vi "Practica02.vi"() -> ()   [LabVIEW 2021]
uses:
  <vilib>/DAQmx/configure/timing.llb/DAQmx Timing (Sample Clock).vi
  <vilib>/DAQmx/create/channels.llb/DAQmx Create Channel (DI-Digital Input).vi
  <vilib>/DAQmx/read.llb/DAQmx Read (Digital 1D Bool 1Chan 1Samp).vi
  <vilib>/Utility/file.llb/Write Delimited Spreadsheet (DBL).vi
panel:
  out "Numero":u32
  out "appended array":bool[](array[boolean])
  in  "stop":bool
  out "Slide":dbl(slide) scale=0.0..1.0
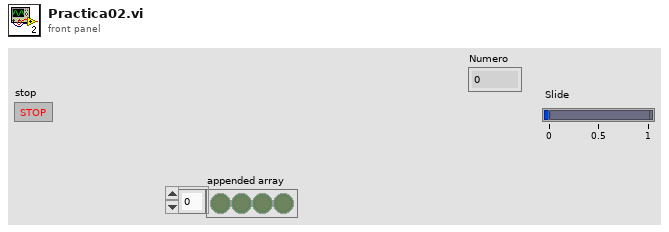
[diagram p1: front panel]
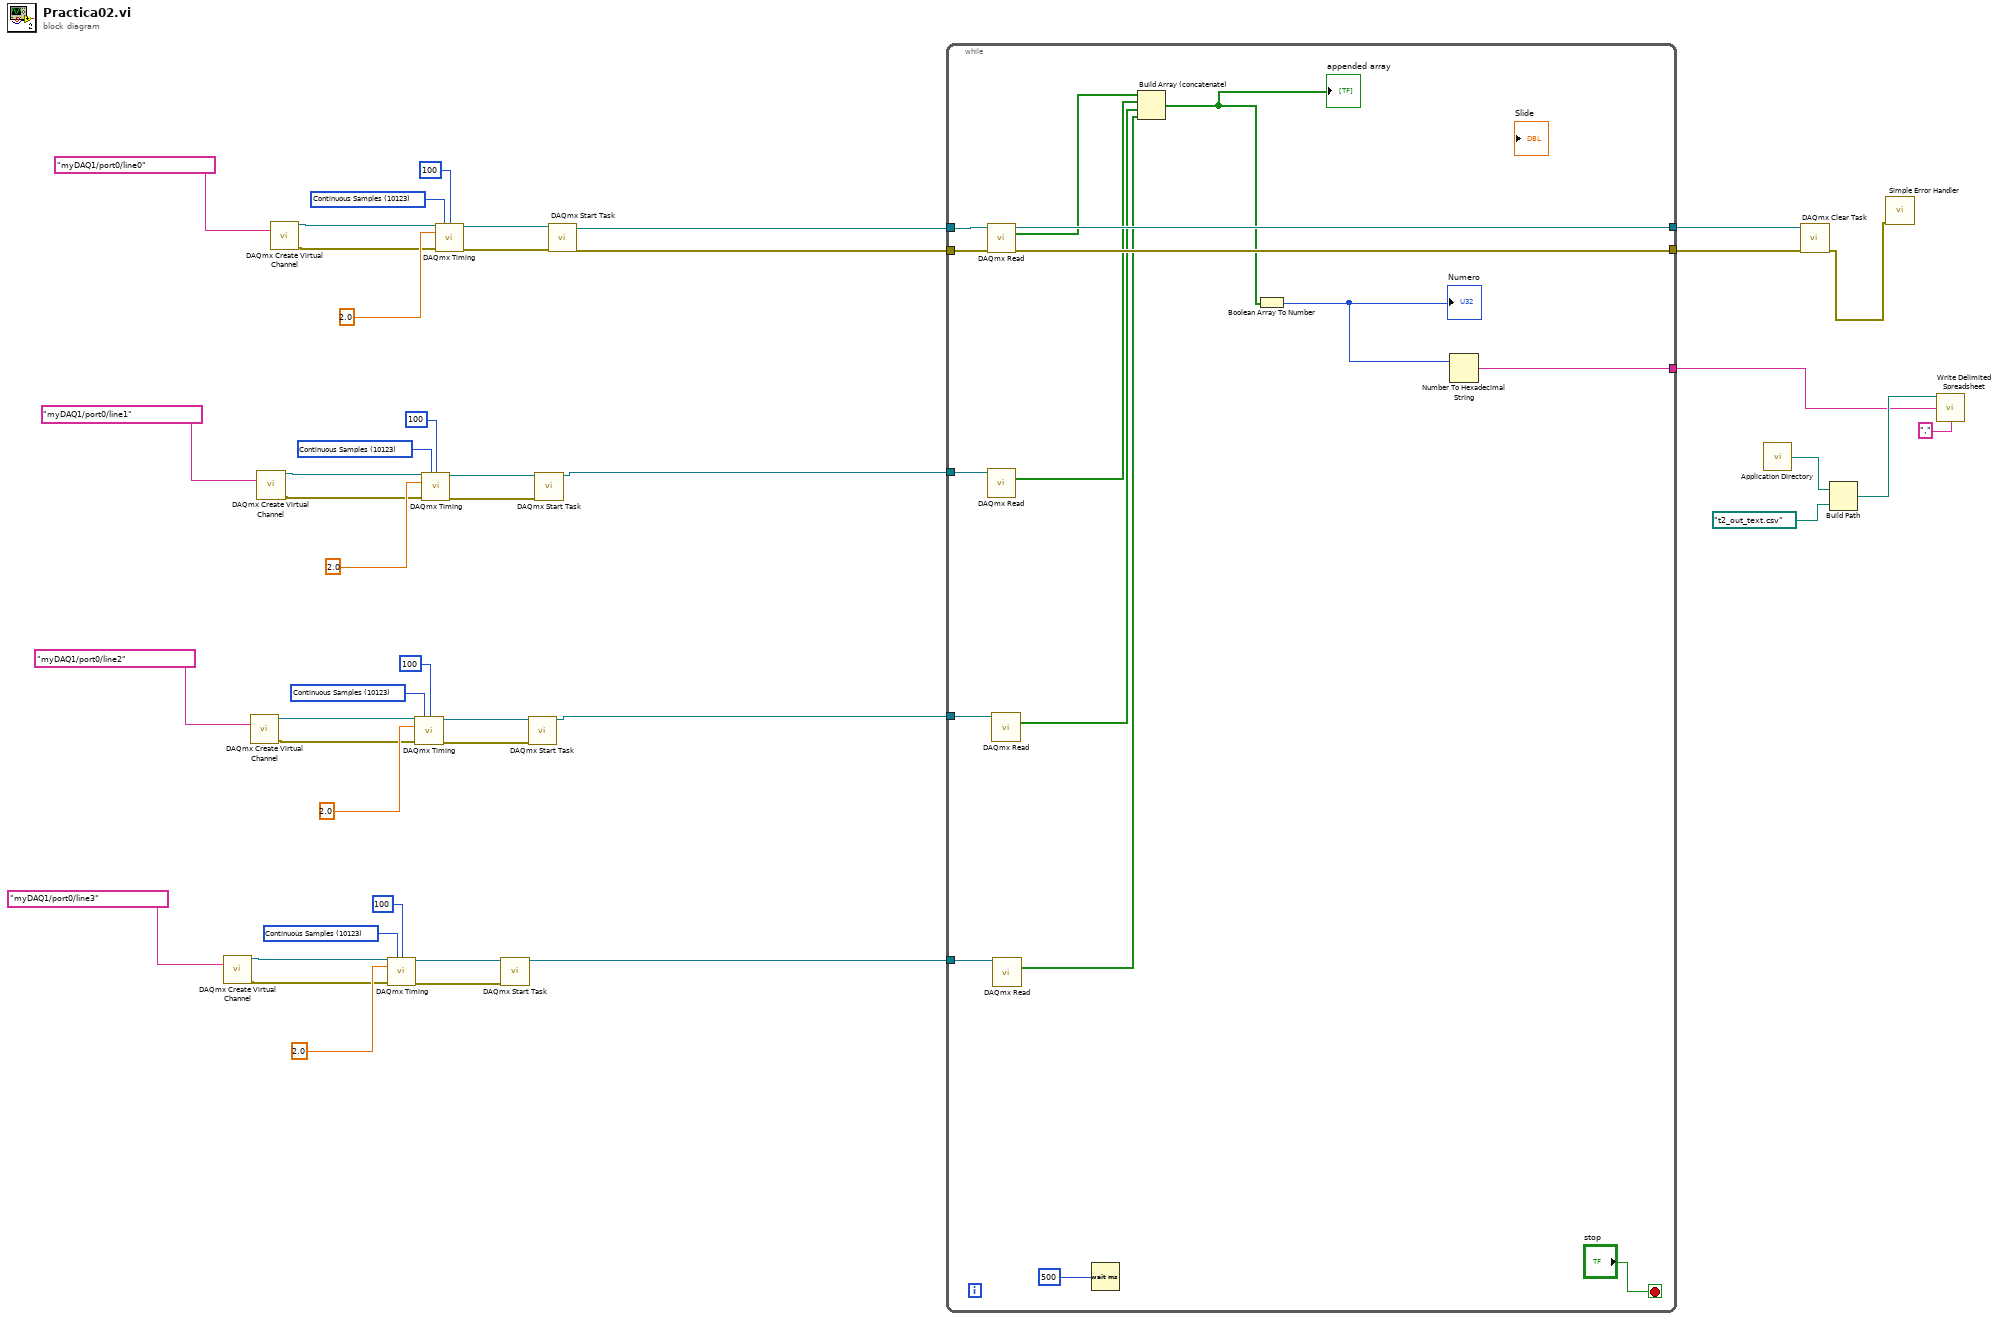
[diagram p0: block diagram]
diagram:
  w16 = 10123 items=["Finite Samples"=10178, "Continuous Samples"=10123, "Hardware Timed Single Point"=12522] ("sample mode")
  w24 = 10123 items=["Finite Samples"=10178, "Continuous Samples"=10123, "Hardware Timed Single Point"=12522] ("sample mode")
  w32 = 10123 items=["Finite Samples"=10178, "Continuous Samples"=10123, "Hardware Timed Single Point"=12522] ("sample mode")
  w45 = 10123 items=["Finite Samples"=10178, "Continuous Samples"=10123, "Hardware Timed Single Point"=12522] ("sample mode")
  n1 = call-poly <vilib>:"DAQmx Create Virtual Channel.vi"("lines"=tag "myDAQ1/port0/line3") -> ("task out"=w11:refnum<k21>, "error out"=w10:errorcluster)  [unwired: 13 in]
  n2 = call-poly <vilib>:"DAQmx Create Virtual Channel.vi"("lines"=tag "myDAQ1/port0/line2") -> ("task out"=w19:refnum<k21>, "error out"=w18:errorcluster)  [unwired: 13 in]
  n3 = call-poly <vilib>:"DAQmx Create Virtual Channel.vi"("lines"=tag "myDAQ1/port0/line1") -> ("task out"=w27:refnum<k21>, "error out"=w26:errorcluster)  [unwired: 13 in]
  n4 = call-poly <vilib>:"DAQmx Create Virtual Channel.vi"("lines"=tag "myDAQ1/port0/line0") -> ("task out"=w35:refnum<k21>, "error out"=w34:errorcluster)  [unwired: 13 in]
  n5 = call-poly <vilib>:"DAQmx Timing.vi"("task/channels in"=w11, "sample mode"=w16, "samples per channel"=100, "rate"=2.0, "error in"=w10) -> ("task out"=w13:refnum<k21>, "error out"=w12:errorcluster)  [unwired: 9 in]
  n6 = call-poly <vilib>:"DAQmx Timing.vi"("task/channels in"=w19, "sample mode"=w24, "samples per channel"=100, "rate"=2.0, "error in"=w18) -> ("task out"=w21:refnum<k21>, "error out"=w20:errorcluster)  [unwired: 9 in]
  n7 = call-poly <vilib>:"DAQmx Timing.vi"("task/channels in"=w27, "sample mode"=w32, "samples per channel"=100, "rate"=2.0, "error in"=w26) -> ("task out"=w29:refnum<k21>, "error out"=w28:errorcluster)  [unwired: 9 in]
  n8 = call-poly <vilib>:"DAQmx Timing.vi"("task/channels in"=w35, "sample mode"=w45, "samples per channel"=100, "rate"=2.0, "error in"=w34) -> ("task out"=w42:refnum<k21>, "error out"=w41:errorcluster)  [unwired: 9 in]
  n9 = call <vilib>:"DAQmx Start Task.vi"("task/channels in"=w13, "error in"=w12) -> ("task out"=w6:refnum<k21>)  [unwired: 12 in, 1 out]
  n10 = call <vilib>:"DAQmx Start Task.vi"("task/channels in"=w21, "error in"=w20) -> ("task out"=w7:refnum<k21>)  [unwired: 12 in, 1 out]
  n11 = call <vilib>:"DAQmx Start Task.vi"("task/channels in"=w29, "error in"=w28) -> ("task out"=w8:refnum<k21>)  [unwired: 12 in, 1 out]
  n12 = call <vilib>:"DAQmx Start Task.vi"("task/channels in"=w42, "error in"=w41) -> ("task out"=w40:refnum<k21>, "error out"=w39:errorcluster)  [unwired: 12 in]
  n13 = while {
    tunnel: w40 -> [w61]
    tunnel: w39 -> [w60]
    tunnel: [w59] -> w38
    tunnel: [w58] -> w37
    tunnel: w8 -> [w56]
    tunnel: w7 -> [w55]
    tunnel: w6 -> [w54]
    tunnel: [w46] -> w1
    stop <- "stop" stop-if-true
    n14 = call-poly <vilib>:"DAQmx Read.vi"("task/channels in"=w61, "error in"=w60) -> ("task out"=w59:refnum<k21>, "data"=w52:bool[], "error out"=w58:errorcluster)  [unwired: 11 in]
    n15 = call-poly <vilib>:"DAQmx Read.vi"("task/channels in"=w56) -> ("data"=w51:bool[])  [unwired: 12 in, 2 out]
    n16 = call-poly <vilib>:"DAQmx Read.vi"("task/channels in"=w55) -> ("data"=w50:bool[])  [unwired: 12 in, 2 out]
    n17 = call-poly <vilib>:"DAQmx Read.vi"("task/channels in"=w54) -> ("data"=w49:bool[])  [unwired: 12 in, 2 out]
    n18 = Wait (ms)(milliseconds to wait=500) -> ()  [unwired: 1 out]
    n19 = Build Array (concatenate) "Build Array"(w52, w51, w50, w49) -> (w48:bool[])
    "appended array" <- w48
    n20 = Boolean Array To Number(Boolean array=w48) -> (number=w47:u32)
    "Numero" <- w47
    n21 = Number To Hexadecimal String(2:w47) -> (0:w46:string)  [unwired: 1 in]
  }
  n22 = call <vilib>:"Application Directory.vi"() -> ("Application Directory"=w5:path)
  n23 = call <vilib>:"DAQmx Clear Task.vi"("task in"=w38, "error in"=w37) -> ("error out"=w36:errorcluster)  [unwired: 13 in]
  n24 = Build Path(base path=w5, name or relative path=path "t2_out_text.csv" ("file (use dialog)")) -> (appended path=w3:path)
  n25 = call <vilib>:"Simple Error Handler.vi"("error in (no error)"=w36) -> ()  [unwired: 4 in, 5 out]
  n26 = call-poly <vilib>:"Write Delimited Spreadsheet.vi"("file path (dialog if empty)"=w3, "1D data"=w1, "delimiter (\\t)"="," ("delimiter (\\t)")) -> ()  [unwired: 11 in, 2 out]
